vi "Generate Unified Msg Set.vi"(11 "Base Actor in":refnum<class "Base Actor.lvclass">) -> (2 "Unified Msg Set":T1)   [LabVIEW 2020, in "jettl.lvlib" / "Actor.lvlib" / "Base Actor.lvclass"]
uses:
  Base Actor.lvclass
  Msg Set.ctl
  Msg/Msg.lvclass
  Actor.lvlib
  C:/git/jettl/src/jettl/jettl/Actor/Base Actor/Base Actor.lvclass
  C:/git/jettl/src/jettl/jettl/Actor/Actor/Actor.lvclass
  C:/git/jettl/src/jettl/jettl/Go To Destroy Msg/Go To Destroy/Go To Destroy.lvclass
  C:/git/jettl/src/jettl/jettl/Has Destroyed Msg/Has Destroyed/Has Destroyed.lvclass
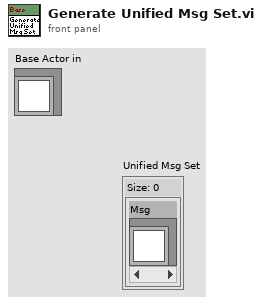
[diagram p1: front panel]
types:
  T1 = typedef "jettl.lvlib/Actor.lvlib/Msg Set.ctl" = set{refnum<class "Msg.lvclass">}
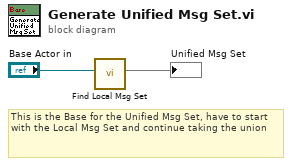
[diagram p0: block diagram]
diagram:
  # "This is the Base for the Unified Msg Set, have to start with the Local Msg Set and continue taking the union"
  n1 = call "Find Local Msg Set.vi"("Actor"="Base Actor in") -> ("Local Msg Set"=→"Unified Msg Set":T1)  [unwired: 10 in]
